vi "Test.vi"() -> ()   [LabVIEW 2013]
uses:
  <vilib>/Instr/_visa.llb/VISA Configure Serial Port (Instr).vi
panel:
  out "String out":string="PHYSIK INSTRUMENTE (PI),Hexapod,0,V6.0.8F 050209900\n0"
  out "error out":errorcluster
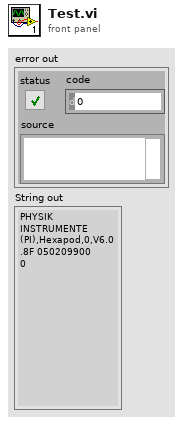
[diagram p1: front panel]
types:
  T1 = cluster{"connection ID":refnum<k5>, "VISA resource name out":refnum<visa-resource-name>, "connectiontype":enum16{"TCPIP", "Serial"}}
  T2 = cluster{"connection ID":refnum<k5>, "VISA resource name":refnum<visa-resource-name>, "Selector":enum16{"TCPIP", "Serial"}}
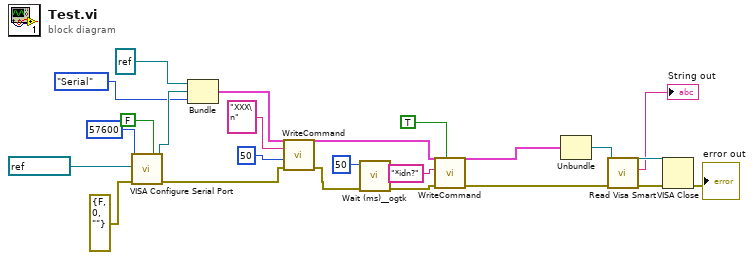
[diagram p0: block diagram]
diagram:
  n1 = call-poly "VISA Configure Serial Port"("VISA resource name"=refnum<visa-resource-name> "COM1", "Enable Termination\nChar (T)"=FALSE ("Enable Termination\nChar (T)"), "baud rate (9600)"=u32 57600, "error in (no error)"=errorcluster {"status"=FALSE, "code"=0, "source"=""}) -> ("VISA resource name out"=w19:refnum<visa-resource-name>, "error out"=w4:errorcluster)  [unwired: 10 in]
  n2 = Bundle("connection ID"=refnum<k5> refnum, "VISA resource name out"=w19, "connectiontype"=enum16{"TCPIP", "Serial"}."Serial") -> (w6:T1)  [unwired: 1 in]
  n3 = call "WriteCommand.vi"("error in (no error)"=w4, "timeout ms (0)"=50, "String"="XXX\n" ("Interface clear"), "Connection"=w6) -> ("error out"=w3:errorcluster, "Connection out"=w5:T2)  [unwired: 6 in]
  n4 = call <userlib>:"Wait (ms)__ogtk.vi"("error in (no error)"=w3, "milliseconds to wait"=u32 50) -> ("error out"=w2:errorcluster)  [unwired: 8 in, 1 out]
  n5 = call "WriteCommand.vi"("Attach Linefeed"=TRUE, "error in (no error)"=w2, "String"="*idn?" ("String to Send"), "Connection"=w5) -> ("error out"=w10:errorcluster, "Connection out"=w14:T2)  [unwired: 6 in]
  n6 = Unbundle(w14) -> ("VISA resource name"=w13:refnum<visa-resource-name>)  [unwired: 2 out]
  n7 = call "Read Visa Smart.vi"("error in (no error)"=w10, "VISA Refnum in"=w13) -> ("error out"=w11:errorcluster, "String"=→"String out":string, "VISA Refnum out"=w12:refnum<visa-resource-name>)  [unwired: 7 in]
  n8 = VISA Close(VISA resource name=w12, error in (no error)=w11) -> (error out=→"error out":errorcluster)
